vi "PXI-Wait for Fresh AI Data Bank.vi"(8 "error in (no error)":errorcluster, 10 "timeout (ms)":i32=5000) -> (0 "error out":errorcluster={"status"=TRUE, "code"=555, "source"="Timed out waiting for Signal Bank."}, 2 "Time":i32)   [LabVIEW 2020]
uses:
  PXI Globals.vi
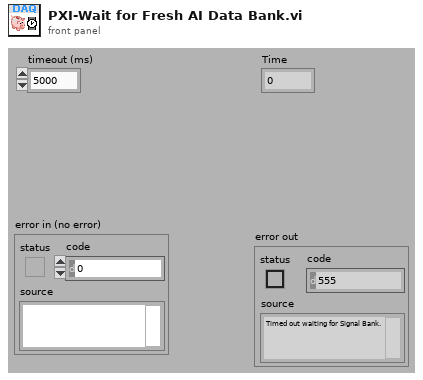
[diagram p1: front panel]
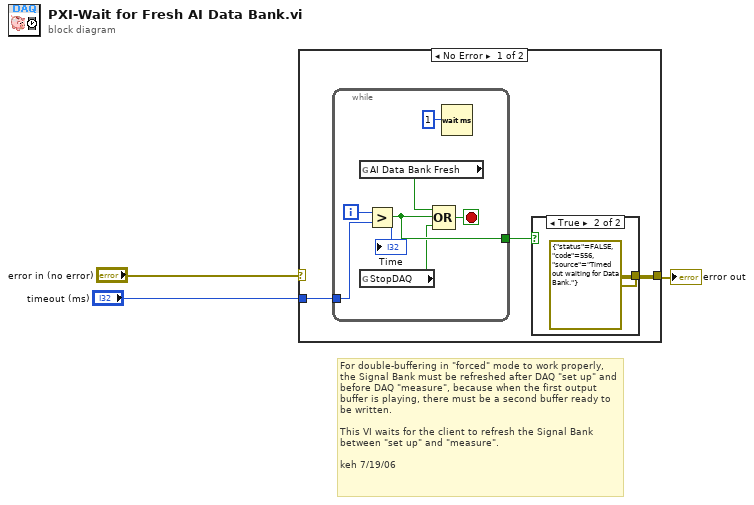
[diagram p0: block diagram]
diagram:
  # "For double-buffering in \"forced\" mode to work properly, the Signal Bank must be refreshed after DAQ \"set up\" and before DAQ \"measure\", because when the first output buffer is playing, there must be a second buffer ready to be written. \n\nThis VI waits for the client to refresh the Signal Bank between \"set up\" and \"measure\".\n\nkeh 7/19/06"
  n1 = case shown="No Error" "error in (no error)" {
    selector: "error in (no error)" -> [_ w15]
    tunnel: [w5 w15] -> w3
    tunnel: "timeout (ms)" -> [w4 _]
    frame No Error {
      n2 = while {
        tunnel: w4 -> [w10]
        tunnel: [w11] -> w6
        i -> [w12]
        stop <- w13 stop-if-true
        n3 = global read "PXI Globals.vi" "AI Data Bank Fresh"() -> (w8:bool)
        n4 = global read "PXI Globals.vi" "StopDAQ"() -> (w9:bool)
        n5 = Greater?(x=w12, y=w10) -> (0:w11:bool)
        n6 = Compound Arithmetic op=OR(w8, w11, w9) -> (w13:bool)
        n7 = Wait (ms)(milliseconds to wait=1) -> ()  [unwired: 1 out]
        "Time" <- w12
      }
      n8 = case shown="True" w6 {
        tunnel: [_ errorcluster {"status"=FALSE, "code"=556, "source"="Timed out waiting for Data Bank."} ("error out 2")] -> w5
        frame False {
        }
        frame True {
        }
      }
    }
    frame Error {
    }
  }
  "error out" <- w3
